vi "TaskControl Page.vi"(8 "?":errorcluster) -> ()   [LabVIEW 2020, in "Vires VTD System Explorer.lvlib"]
uses:
  Vires VTD System Explorer.lvlib
  <vilib>/NI VeriStand/Custom Device API/Custom Device Item Ref.ctl
  Shared/Network Settings.ctl
  Shared/Protocol.ctl
  <vilib>/NI VeriStand/Custom Device API/Custom Device API.lvlib
  Shared/Vires VTD Shared.lvlib
panel:
  in  "Network Settings":T1={"IP adress"="", "RDB"={"Protocol"=enum."UDP", "Tx Port"=48191, "Rx Port"=48191, "Buffer Size"=204800, "Timeout"=10}, "SCP"={"Protocol"=enum."TCP", "Tx Port"=48191, "Rx Port"=48191, "Buffer Size"=204800, "Timeout"=10}}
  in  "Header 2":cluster{"Section Name":string}={"Section Name"="Task Control Network Settings"}
  in  "Header":cluster{"Section Name":string}={"Section Name"="Custom Device Item Settings"}
  in  "Description":string
  in  "Name":string
  in  "Node Ptr":T3 format="%.0x"
  out "error out":errorcluster
  in  "SHDocVw.IWebBrowser2":refnum<k7>(container)
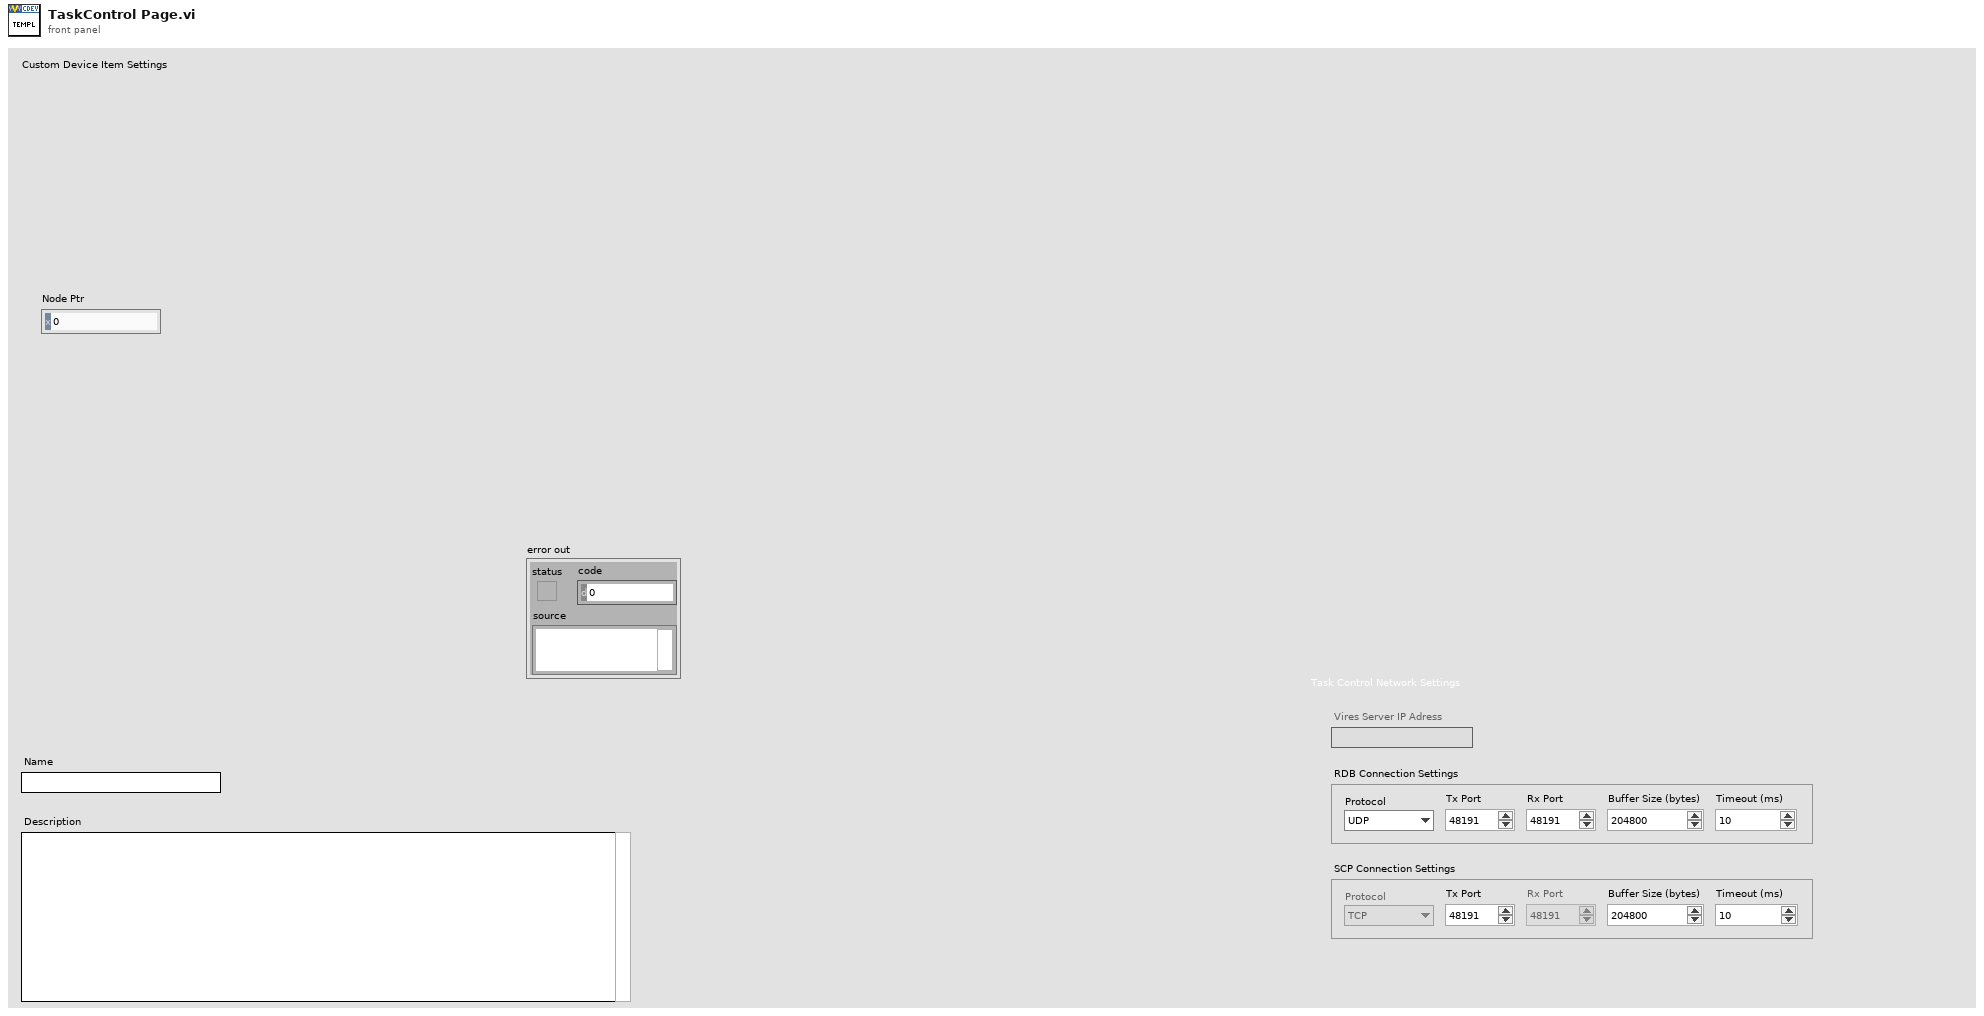
[diagram p1: front panel]
types:
  T1 = typedef "Vires VTD Shared.lvlib/Network Settings.ctl" = cluster{"IP adress":string, "RDB":cluster{"Protocol":T2, "Tx Port":u16, "Rx Port":u16, "Buffer Size":i32, "Timeout":u16}, "SCP":cluster{"Protocol":T2, "Tx Port":u16, "Rx Port":u16, "Buffer Size":i32, "Timeout":u16}}
  T2 = typedef "Vires VTD Shared.lvlib/Protocol.ctl" = enum16{"UDP", "TCP"}
  T3 = typedef "Custom Device API.lvlib/Custom Device Item Ref.ctl" = u64
  T4 = enum8{"Enabled", "Disabled", "Disabled and Grayed Out"}
  T5 = typedef "Custom Device API.lvlib/Custom Device Item Info.ctl" = cluster{"Name":string, "Is Channel":bool, "GUID":string, "Is Waveform":bool}
  T6 = typedef "Custom Device API.lvlib/Custom Device Commands.ctl" = enum16{"Default", "Item renamed", "Shutdown", "Dynamic button pressed"}
  T7 = cluster{"Protocol":T2, "Tx Port":u16, "Rx Port":u16, "Buffer Size":i32, "Timeout":u16}
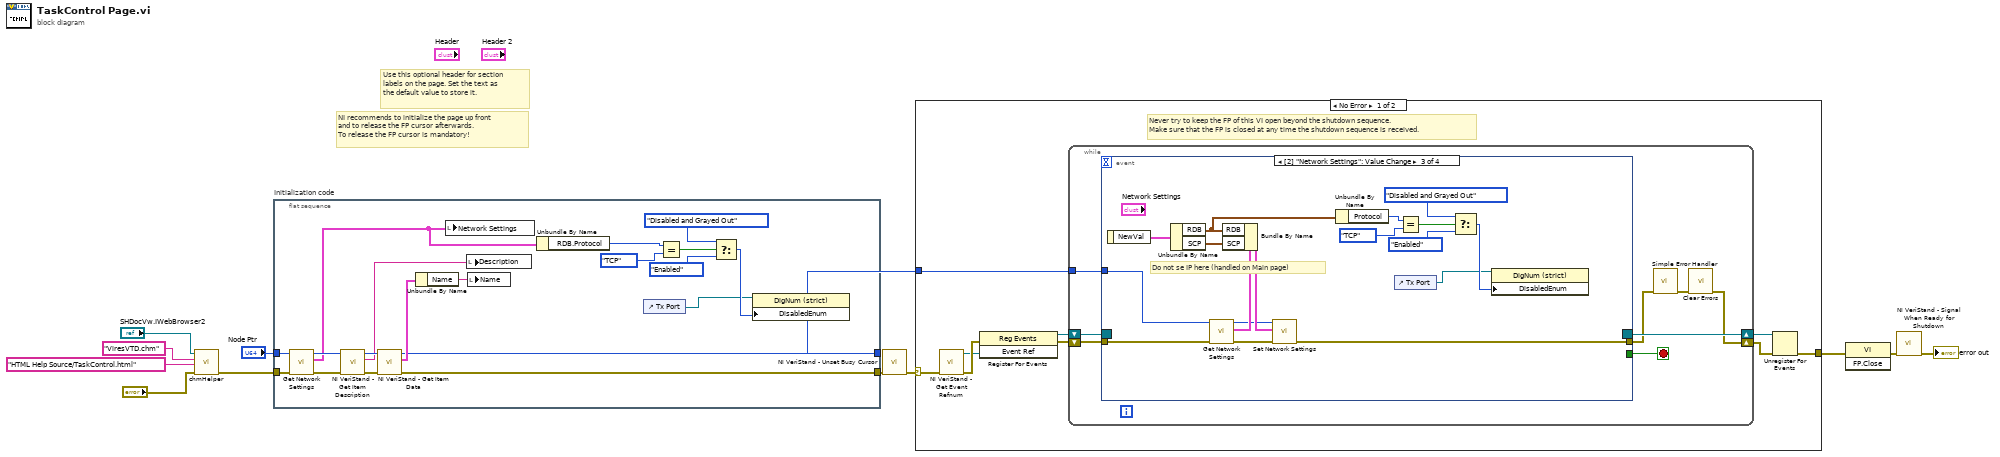
[diagram p0: block diagram]
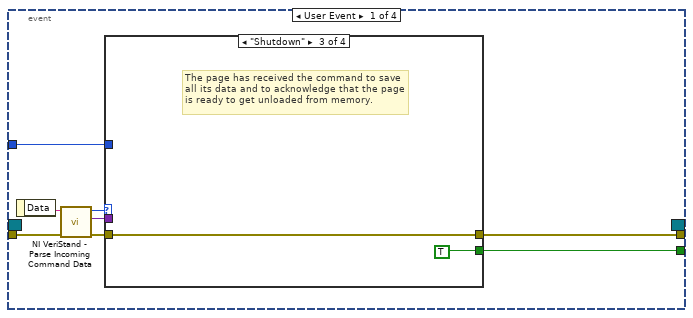
[diagram p2: hidden frame]
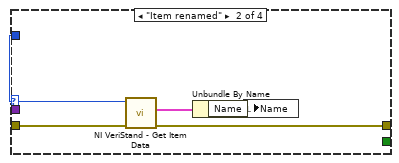
[diagram p4: hidden frame]
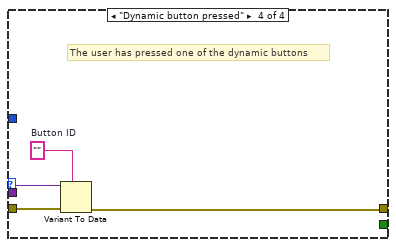
[diagram p5: hidden frame]
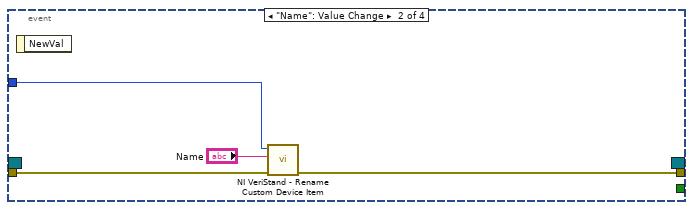
[diagram p6: hidden frame]
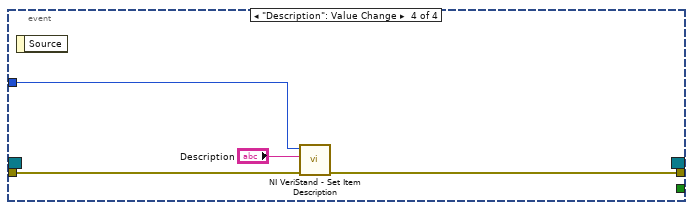
[diagram p7: hidden frame]
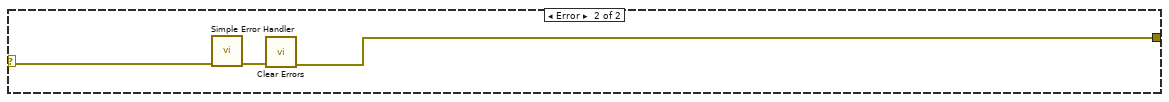
[diagram p8: hidden frame]
diagram:
  # "Use this optional header for section labels on the page. Set the text as the default value to store it."
  # "NI recommends to initialize the page up front\nand to release the FP cursor afterwards.\nTo release the FP cursor is mandatory!"
  n1 = call "chmHelper.vi"("error in (no error)"="?", "HTML File"="HTML Help Source/TaskControl.html", "Main CHM File"="ViresVTD.chm" ("HTML File"), "Automation Refnum in"="SHDocVw.IWebBrowser2") -> ("error out"=w2:errorcluster)  [unwired: 7 in]
  n2 = flat-sequence "Initialization code" {
    tunnel: "Node Ptr" -> [w25]
    tunnel: [w26] -> w8
    tunnel: w2 -> [w24]
    tunnel: [w21] -> w1
    frame #0 {
      n3 = call "Get Network Settings.vi"("error in"=w24, "Item Ref in"=w25) -> ("error out"=w23:errorcluster, "Network Settings"=w20:T1, "Item Ref out"=w22:T3)  [unwired: 7 in]
      n4 = call <vilib>:"NI VeriStand - Get Item Description.vi"("error in (no error)"=w23, "Item Ref in"=w22) -> ("error out"=w29:errorcluster, "Description"=w30:string, "Item Ref out"=w31:T3)  [unwired: 7 out]
      n5 = call <vilib>:"NI VeriStand - Get Item Data.vi"("error in (no error)"=w29, "Item Ref in"=w31) -> ("error out"=w21:errorcluster, "Item Info"=w28:T5, "Item Ref out"=w26:T3)  [unwired: 7 out]
      n6 = Unbundle By Name(w28) -> ("Name"=w27:string)
      n7 = local write "Network Settings"(w20) -> ()
      n8 = local write "Description"(w30) -> ()
      n9 = local write "Name"(w27) -> ()
      n10 = Unbundle By Name(w20) -> ("RDB.Protocol"=w14:T2)
      n11 = control-ref of="Tx Port"() -> (w13:refnum<vi>)
      n12 = Equal?(x=w14, y=Protocol."TCP") -> (x = y?=w18:bool)
      n13 = Select(t=T4."Disabled and Grayed Out" ("Disabled"), s=w18, f=T4."Enabled" ("Disabled")) -> (s? t:f=w17:T4)
      n14 = property class="DigNum (strict)"(reference=w13, "DisabledEnum"=w17) -> ()  [unwired: 1 in, 2 out]
    }
  }
  n15 = call <vilib>:"NI VeriStand - Unset Busy Cursor.vi"("error in (no error)"=w1) -> ("error out"=w9:errorcluster)  [unwired: 10 out]
  n16 = case shown="No Error" w9 {
    selector: w9 -> [w32 w96]
    tunnel: [w37 w94] -> w12
    tunnel: w8 -> [w33 _]
    frame No Error {
      # "Never try to keep the FP of this VI open beyond the shutdown sequence.\nMake sure that the FP is closed at any time the shutdown sequence is received."
      n17 = call <vilib>:"NI VeriStand - Get Event Refnum.vi"("error in (no error)"=w32) -> ("error out"=w40:errorcluster, "Event Ref"=w36:refnum<user-event>)  [unwired: 9 out]
      n18 = register-events(error in=w40, w36) -> (reference out=w34:refnum<event-registration>, error out=w35:errorcluster)  [unwired: 1 in]
      n19 = while {
        tunnel: w33 -> [w44]
        shift-right: [w41] -> w38
        shift-left: w35 -> [w47]
        shift-right: [w48] -> w39
        shift-left: w34 -> [w46]
        stop <- w45 stop-if-true
        n20 = event shown="[2] \"Network Settings\": Value Change" {
          selector: w46 -> [_ _ _ _]
          dyn-events: [_ _ _ _] -> w48
          timeout: _ -> [_ _ _ _]
          tunnel: w47 -> [w56 w72 w86 w92]
          tunnel: [w52 _ _ _] -> w45
          tunnel: [w51 w71 w85 w91] -> w43
          tunnel: w44 -> [w50 w70 w84 w93]
          event User Event {
            n21 = event-data() -> ("Data"=w55:string)  [unwired: 1 out]
            n22 = call <vilib>:"NI VeriStand - Parse Incoming Command Data.vi"("error in (no error)"=w56, "Incoming data"=w55) -> ("error out"=w54:errorcluster, "Outgoing data"=w49:variant, "Action"=w53:T6)  [unwired: 7 out]
            n23 = case shown="\"Shutdown\"" w53 {
              tunnel: w54 -> [w57 w62 w63 w68]
              tunnel: [_ _ TRUE _] -> w52
              tunnel: [w57 w60 w63 w65] -> w51
              tunnel: w50 -> [_ w58 _ _]
              tunnel: w49 -> [_ _ _ w67]
              frame "Default", Default {
              }
              frame "Item renamed" {
                n24 = call <vilib>:"NI VeriStand - Get Item Data.vi"("error in (no error)"=w62, "Item Ref in"=w58) -> ("error out"=w60:errorcluster, "Item Info"=w61:T5)  [unwired: 8 out]
                n25 = Unbundle By Name(w61) -> ("Name"=w59:string)
                n26 = local write "Name"(w59) -> ()
              }
              frame "Shutdown" {
                # "The page has received the command to save all its data and to acknowledge that the page is ready to get unloaded from memory."
              }
              frame "Dynamic button pressed" {
                w66 = ""  # Button ID
                # "The user has pressed one of the dynamic buttons"
                n27 = Variant To Data(error in=w68, type=w66, Variant=w67) -> (error out=w65:errorcluster)  [unwired: 1 out]
              }
            }
          }
          event "Name": Value Change {
            n28 = event-data() -> ()  [unwired: 2 out]
            n29 = call <vilib>:"NI VeriStand - Rename Custom Device Item.vi"("error in (no error)"=w72, "New Name"="Name", "Item Ref in"=w70) -> ("error out"=w71:errorcluster)  [unwired: 1 in, 7 out]
          }
          event Value Change {
            # "Do not se IP here (handled on Main page)"
            n30 = event-data() -> ("NewVal"=w83:T1)  [unwired: 1 out]
            n31 = Unbundle By Name(w83) -> ("RDB"=w80:T7, "SCP"=w82:T7)
            n32 = call "Get Network Settings.vi"("error in"=w86, "Item Ref in"=w84) -> ("error out"=w81:errorcluster, "Network Settings"=w88:T1, "Item Ref out"=w87:T3)  [unwired: 7 in]
            n33 = Bundle By Name(cluster=w88, "RDB"=w80, "SCP"=w82) -> (w89:T1)
            n34 = call "Set Network Settings.vi"("error in"=w81, "Network Settings"=w89, "Item Ref in"=w87) -> ("error out"=w85:errorcluster)  [unwired: 7 in, 1 out]
            n35 = Unbundle By Name(w80) -> ("Protocol"=w79:T2)
            n36 = control-ref of="Tx Port"() -> (w73:refnum<vi>)
            n37 = Equal?(x=w79, y=Protocol."TCP") -> (x = y?=w77:bool)
            n38 = Select(t=T4."Disabled and Grayed Out" ("Disabled"), s=w77, f=T4."Enabled" ("Disabled")) -> (s? t:f=w76:T4)
            n39 = property class="DigNum (strict)"(reference=w73, "DisabledEnum"=w76) -> ()  [unwired: 1 in, 2 out]
          }
          event "Description": Value Change {
            n40 = event-data() -> ()  [unwired: 2 out]
            n41 = call <vilib>:"NI VeriStand - Set Item Description.vi"("error in (no error)"=w92, "Description"="Description", "Item Ref in"=w93) -> ("error out"=w91:errorcluster)  [unwired: 8 out]
          }
        }
        n42 = call <vilib>:"Simple Error Handler.vi"("error in (no error)"=w43) -> ("error out"=w42:errorcluster)  [unwired: 1 in, 7 out]
        n43 = call <vilib>:"Clear Errors.vi"("error in (no error)"=w42) -> ("error out"=w41:errorcluster)  [unwired: 1 in, 5 out]
      }
      n44 = Unregister For Events(event registration refnum=w39, error in=w38) -> (error out=w37:errorcluster)
    }
    frame Error {
      n45 = call <vilib>:"Simple Error Handler.vi"("error in (no error)"=w96) -> ("error out"=w95:errorcluster)  [unwired: 1 in, 7 out]
      n46 = call <vilib>:"Clear Errors.vi"("error in (no error)"=w95) -> ("error out"=w94:errorcluster)  [unwired: 1 in, 5 out]
    }
  }
  n47 = invoke class="VI" method="FP.Close"(error in=w12) -> (error out=w11:errorcluster)  [unwired: 2 in, 2 out]
  n48 = call <vilib>:"NI VeriStand - Signal When Ready for Shutdown.vi"("error in (no error)"=w11) -> ("error out"=→"error out":errorcluster)  [unwired: 10 out]
